vi "Tegam4040_Offset_Global.vi"() -> ()   [LabVIEW 2010]
panel:
  in  "Tegam Offsets 100V":cluster{"tegam2_DAC":u16, "tegam1_DAC":u16}={"tegam2_DAC"=32767, "tegam1_DAC"=32767} {"tegam1_DAC" format="%04x"; "tegam2_DAC" format="%04x"}
  in  "Tegam Offsets 10V":cluster{"tegam2_DAC":u16, "tegam1_DAC":u16}={"tegam2_DAC"=32767, "tegam1_DAC"=32767} {"tegam1_DAC" format="%04x"; "tegam2_DAC" format="%04x"}
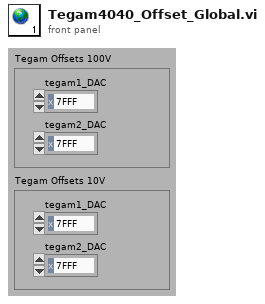
[diagram p1: front panel]
diagram:
